vi "MultipleSignalsGenerator.vi"() -> ()   [LabVIEW 2011]
uses:
  <vilib>/measure/NI_MABase.lvlib
panel:
  out "Waveform Graph":waveform(dbl)(graph)
  out "error out":errorcluster
  in  "Sampling":cluster{"Fs":dbl, " #s":dbl}={"Fs"=1000.0, " #s"=1000.0} {"#s" format="%.2g"; "Fs" format="%.2g"}
  in  "Reset phase":bool
  in  "stop":bool
  in  "Signal Source":T1(ring)
  in  "Phase":dbl format="%.2g"
  in  "Square duty cycle(%)":dbl=50.0 format="%.2g"
  in  "Frequency":dbl=2.0 format="%.2g"
  in  "Amplitude":dbl=1.0 format="%.2g"
  # "ALEXANDRESCU Anda Cristiana\n334 AB\nGenerator de semnale multiple"
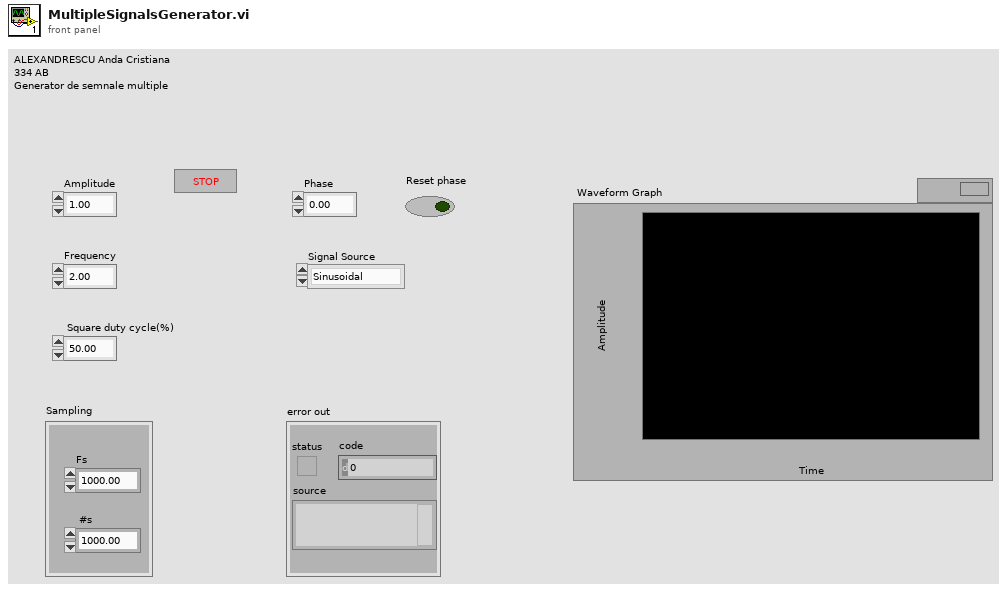
[diagram p1: front panel]
types:
  T1 = enum16{"Sinusoidal", "Dreptunghic", "Dinte de fierastrau", "Triunghiular"}
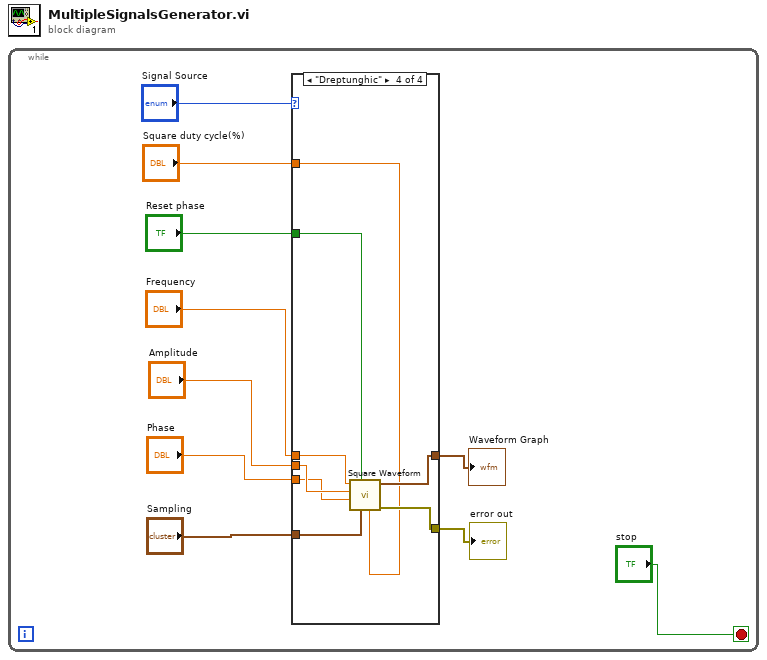
[diagram p0: block diagram]
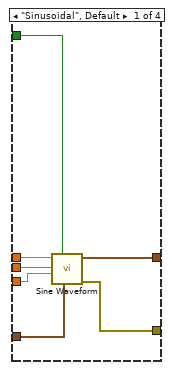
[diagram p2: hidden frame]
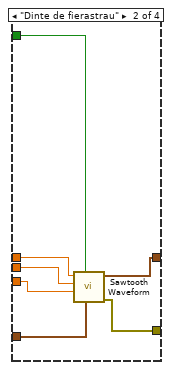
[diagram p3: hidden frame]
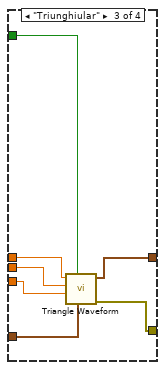
[diagram p4: hidden frame]
diagram:
  n1 = while {
    stop <- "stop" stop-if-true
    n2 = case shown="\"Dreptunghic\"" "Signal Source" {
      tunnel: "Reset phase" -> [w17 w20 w25 w33]
      tunnel: "Frequency" -> [w16 w24 w31 w39]
      tunnel: "Amplitude" -> [w15 w23 w30 w38]
      tunnel: "Phase" -> [w14 w22 w29 w37]
      tunnel: "Sampling" -> [w13 w21 w28 w36]
      tunnel: [w12 w18 w27 w35] -> w3
      tunnel: [w11 w19 w26 w34] -> w2
      tunnel: "Square duty cycle(%)" -> [_ _ _ w32]
      frame "Sinusoidal", Default {
        n3 = call <vilib>:"Sine Waveform.vi"("sampling info"=w13, "reset signal"=w17, "phase"=w14, "amplitude"=w15, "frequency"=w16) -> ("error out"=w12:errorcluster, "signal out"=w11:waveform(dbl))  [unwired: 5 in]
      }
      frame "Dinte de fierastrau" {
        n4 = call <vilib>:"Sawtooth Waveform.vi"("sampling info"=w21, "reset signal"=w20, "phase"=w22, "amplitude"=w23, "frequency"=w24) -> ("error out"=w18:errorcluster, "signal out"=w19:waveform(dbl))  [unwired: 5 in]
      }
      frame "Triunghiular" {
        n5 = call <vilib>:"Triangle Waveform.vi"("sampling info"=w28, "reset signal"=w25, "phase"=w29, "amplitude"=w30, "frequency"=w31) -> ("error out"=w27:errorcluster, "signal out"=w26:waveform(dbl))  [unwired: 5 in]
      }
      frame "Dreptunghic" {
        n6 = call <vilib>:"Square Waveform.vi"("duty cycle (%)"=w32, "sampling info"=w36, "reset signal"=w33, "phase"=w37, "amplitude"=w38, "frequency"=w39) -> ("error out"=w35:errorcluster, "signal out"=w34:waveform(dbl))  [unwired: 4 in]
      }
    }
    "error out" <- w3
    "Waveform Graph" <- w2
  }
